vi "Get pos axis.vi"(8 "error in (no error)":errorcluster, 10 "Axis":i32=1 min=1 max=4, 11 "DelayLineSimulation in":refnum<class "DLEmulate.lvclass">) -> (0 "error out":errorcluster, 2 "Pos":dbl, 3 "DelayLineSimulation out":refnum<class "DLEmulate.lvclass">)   [LabVIEW 2020, in "DLEmulate.lvclass"]
uses:
  DLEmulate.lvclass
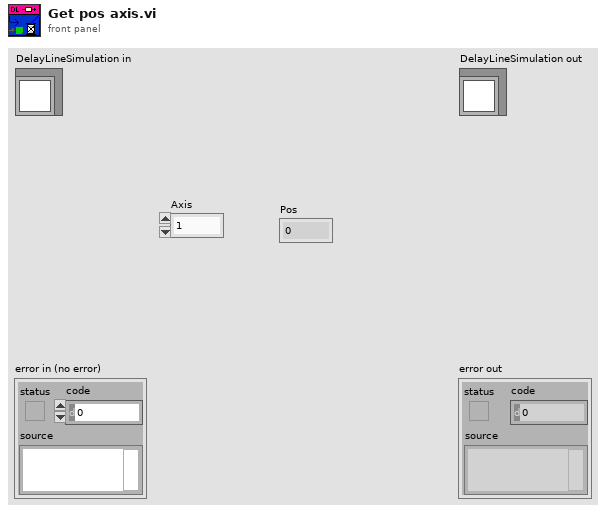
[diagram p1: front panel]
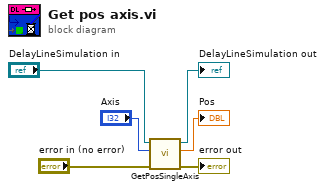
[diagram p0: block diagram]
diagram:
  n1 = call-dynamic "GetPosSingleAxis.vi"("error in (no error)"="error in (no error)", "Axis"="Axis", "DelayLineSimulation in"="DelayLineSimulation in") -> ("error out"=→"error out":errorcluster, "Pos"=→"Pos":dbl, "DelayLineSimulation out"=→"DelayLineSimulation out":refnum<class "DLEmulate.lvclass">)  [unwired: 6 in]
